vi "Update.vi"(8 "error in (no error)":errorcluster, 11 "Generator Base in":refnum<class "Generator Base.lvclass">) -> (0 "error out":errorcluster, 3 "Generator Base out":refnum<class "Generator Base.lvclass">)   [LabVIEW 2018, in "Generator Base.lvlib" / "Generator Base.lvclass"]
uses:
  Generator Base.lvclass
  <vilib>/NI/Event Source Actor/Event Source/Event Source/Event Source.lvclass
  <vilib>/NI/Event Source Actor/Event Source/Event/Event.lvclass
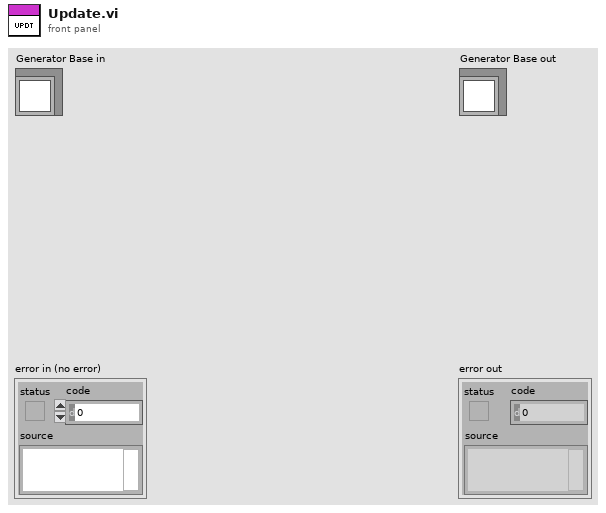
[diagram p1: front panel]
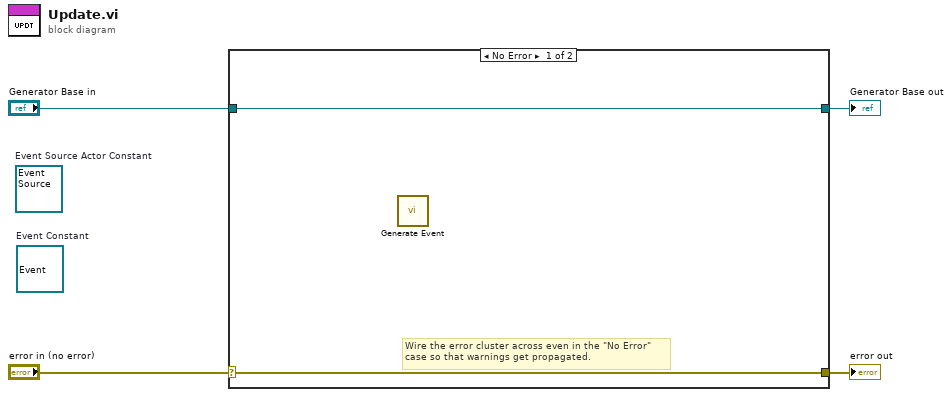
[diagram p0: block diagram]
diagram:
  (unwired) refnum<class "Event.lvclass"> refnum  # Event Constant
  (unwired) refnum<class "Event Source.lvclass"> refnum  # Event Source Actor Constant
  n1 = case shown="No Error" "error in (no error)" {
    selector: "error in (no error)" -> [w5 w8]
    tunnel: [w5 w8] -> w3
    tunnel: [w6 w7] -> w1
    tunnel: "Generator Base in" -> [w6 w7]
    frame No Error {
      # "Wire the error cluster across even in the \"No Error\"\ncase so that warnings get propagated."
      n2 = call <vilib>:"Generate Event.vi"() -> ()  [unwired: 10 in, 2 out]
    }
    frame Error {
    }
  }
  "error out" <- w3
  "Generator Base out" <- w1
